vi "CAN_example_darren.vi"() -> ()   [LabVIEW 2024]
uses:
  <vilib>/Platform/TimedLoop/XDataNode/timing_clust.ctl
  <vilib>/Platform/TimedLoop/XDataNode/nitl_modes.ctl
  <vilib>/Platform/TimedLoop/XDataNode/wakeup.ctl
  <vilib>/addons/Maxon Motor/EPOS2 CANopen/CANopen/sbCANopenBaseClass.lvclass
  <vilib>/platform/TimedLoop/XDataNode/XDataNode.xnode
  <vilib>/Platform/TimedLoop/XDataNode/XDNodeRunTimeDep.lvlib
panel:
  in  "CANcurrent 2":dbl[](array[numeric])
  in  "stop":bool
  out "Write canERROR":errorcluster[](array[cluster])
  out "Write Late":bool
  out "Write Time":i64
  # "Motor Order \n(Trunk, Pelvis, Pelvis_M, Leg)\n3\n6\n9\n12\n2\n7\n8\n13\n4\n5\n10\n11\n1\n14"
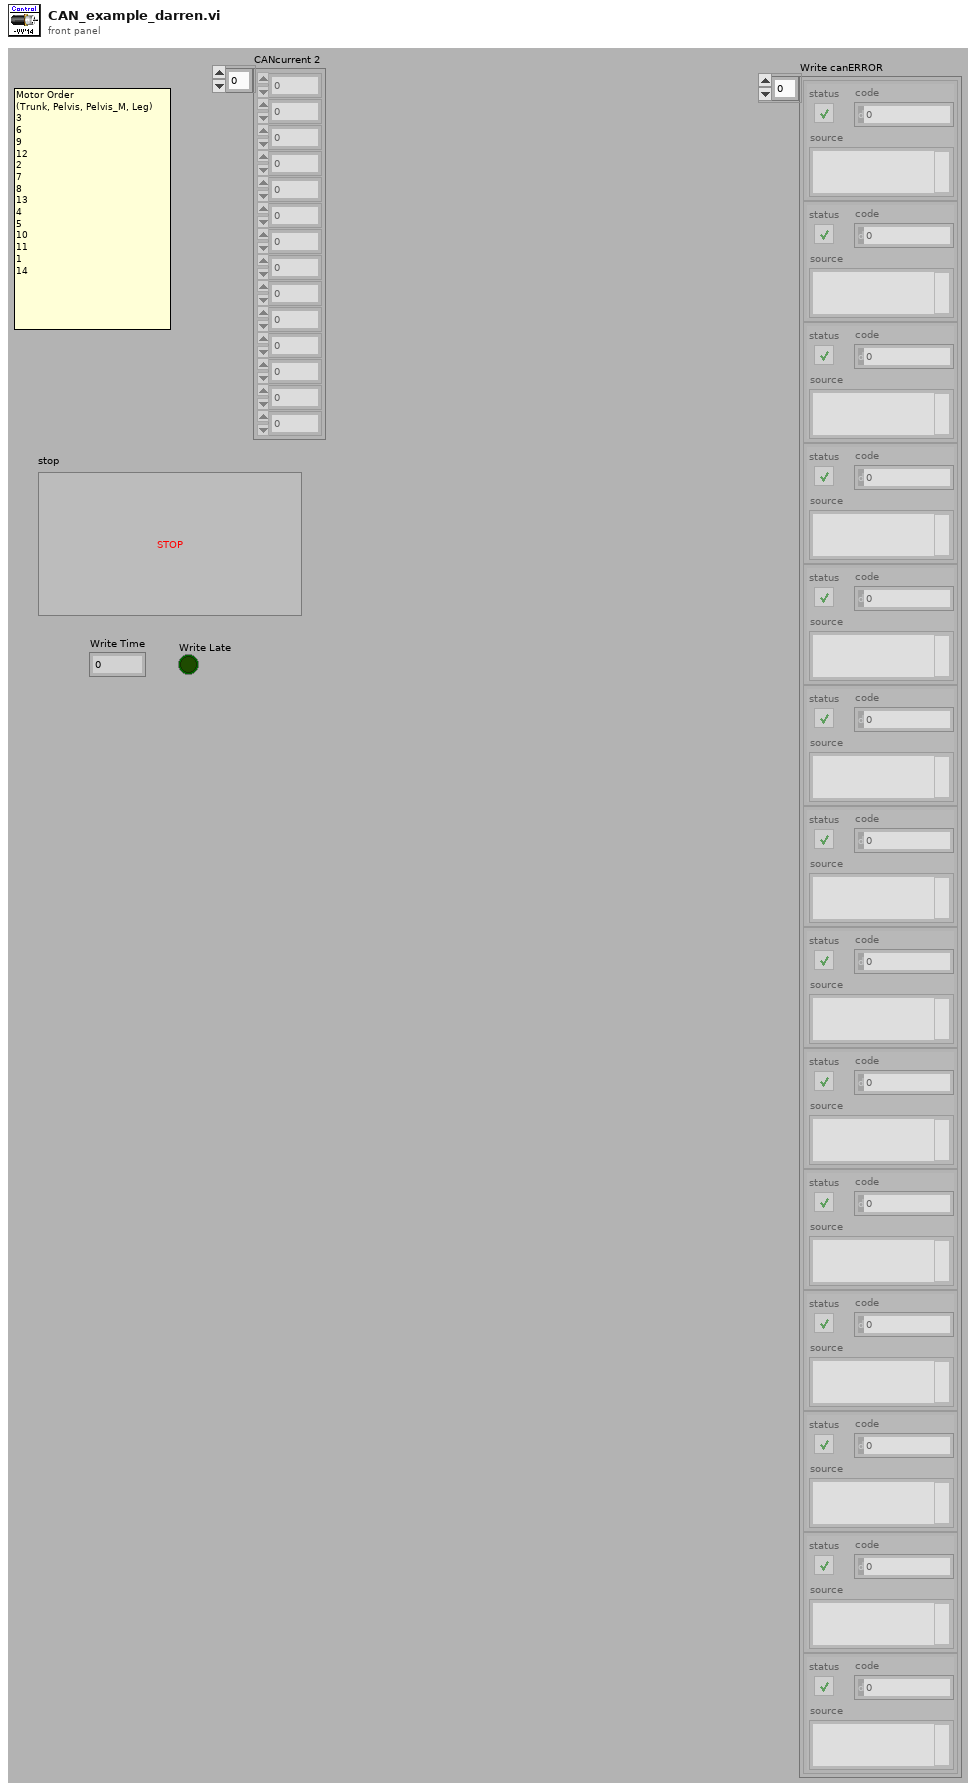
[diagram p1: front panel]
types:
  T1 = typedef "XDNodeRunTimeDep.lvlib/timing_clust.ctl" = cluster{"Expected End [f-1]":u64, "Actual End [f-1]":u64, "Finished Late? [f-1]":bool, "Expected End [i-1]":u64, "Actual End [i-1]":u64, "Finished Late? [i-1]":bool, "Expected Start [i]":u64, "Actual Start [i]":u64, "Expected Start [f]":u64, "Actual Start [f]":u64, "Source Name":string, "Structure Name":string, "Period":i64, "Deadline":i64, "Offset":i64, "Start":i64, "Priority":i32, "Timeout":i32, "Mode":T2, "Wakeup Reason":T3, "Error":errorcluster, "Source Type":string, "Secondary Source Type":string, "Global End Time":u64, "Global Start Time":u64, "Frame Duration":u64, "Iteration Duration":u64, "Assigned CPU":i32, "I/O Scan Engine Mode":u32}
  T2 = typedef "XDNodeRunTimeDep.lvlib/nitl_modes.ctl" = enum32{"No Change", "Process missed periods, maintain original phase", "Discard missed periods, maintain original phase", "Process missed periods, ignore original phase", "Discard missed periods, ignore original phase"}
  T3 = typedef "XDNodeRunTimeDep.lvlib/wakeup.ctl" = enum32{"Normal", "Aborted", "Asynchronous wakeup", "Timing source error", "Timed loop error", "Timeout"}
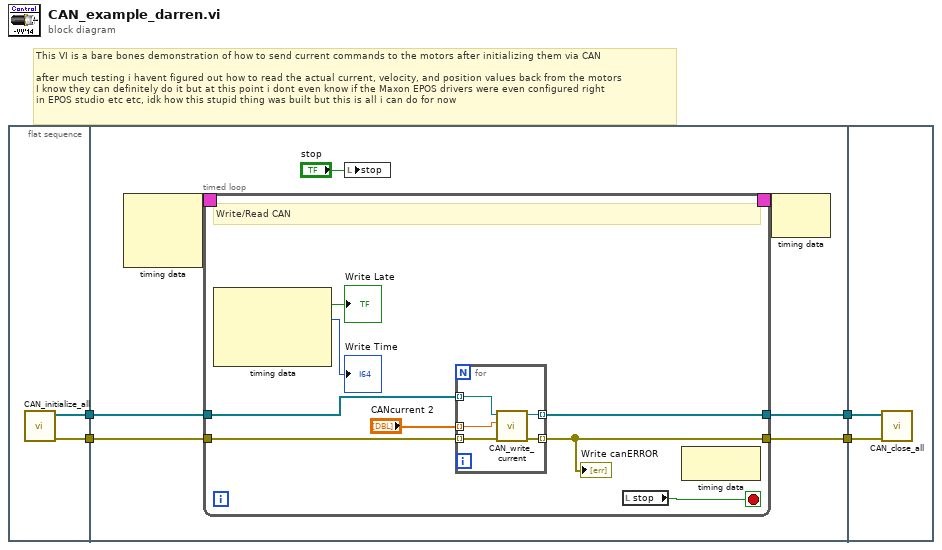
[diagram p0: block diagram]
diagram:
  # "This VI is a bare bones demonstration of how to send current commands to the motors after initializing them via CAN\n\nafter much testing i havent figured out how to read the actual current, velocity, and position values back from the motors\nI know they can definitely do it but at this point i dont even know if the Maxon EPOS drivers were even configured right \nin EPOS studio etc etc, idk how this stupid thing was built but this is all i can do for now"
  n1 = flat-sequence {
    tunnel: [w5] -> w4
    tunnel: [w6] -> w3
    tunnel: w4 -> [w11]
    tunnel: w3 -> [w10]
    tunnel: [w9] -> w2
    tunnel: [w8] -> w1
    tunnel: w2 -> [w34]
    tunnel: w1 -> [w33]
    frame #0 {
      n2 = call "CAN_initialize_all.vi"() -> ("Array of Canopen Sessions"=w6:refnum<class "sbCANopenBaseClass.lvclass">[], "Array of Error out's"=w5:errorcluster[])  [unwired: 5 in]
    }
    frame #1 {
      n3 = node-c288() -> (w13:T1)  [unwired: 3 in]
      n4 = timed-loop {
        tunnel: w11 -> [w19]
        tunnel: [w14] -> w9
        timing: w13 -> [_]
        timing-out: [_] -> w12
        tunnel: w10 -> [w20]
        tunnel: [w15] -> w8
        stop <- w17 stop-if-true
        # "Write/Read CAN"
        n5 = node-c288() -> (→"Write Late":bool, →"Write Time":i64)  [unwired: 1 in, 2 out]
        n6 = for {
          tunnel: [w27] -> w15 mode=indexing
          tunnel: [w28] -> w14 mode=indexing
          tunnel: w20 -> [w29] mode=indexing
          tunnel: w19 -> [w30] mode=indexing
          tunnel: "CANcurrent 2" -> [w26] mode=indexing
          n7 = call "CAN_write_current.vi"("error in"=w30, "Current Command [mA]"=w26, "CANopen Session In"=w29) -> ("error out"=w28:errorcluster, "CANopen Session Out"=w27:refnum<class "sbCANopenBaseClass.lvclass">)  [unwired: 7 in]
        }
        "Write canERROR" <- w14
        n8 = local read "stop"() -> (w17:bool)
        n9 = node-c288() -> ()  [unwired: 1 in, 1 out]
      }
      n10 = local write "stop"("stop") -> ()
      n11 = node-c288(w12) -> ()  [unwired: 1 out]
    }
    frame #2 {
      n12 = call "CAN_close_all.vi"("Input Error out array"=w34, "Input CANopen Sessions array"=w33) -> ()  [unwired: 10 in]
    }
  }
